vi "DAQ - 567 Modules - SubVI.vi"(11 "array":dbl[](array[numeric])) -> (3 "output array":dbl[](array[numeric]))   [LabVIEW 2013]
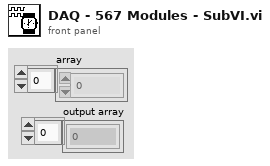
[diagram p1: front panel]
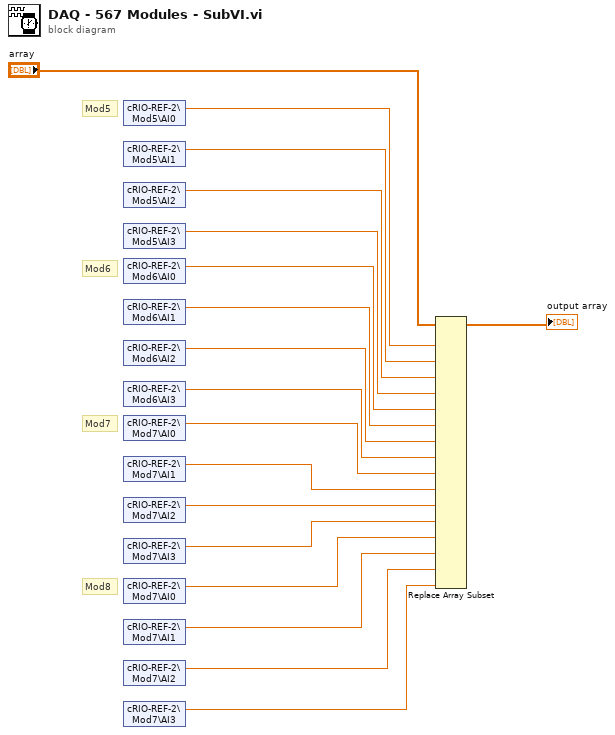
[diagram p0: block diagram]
diagram:
  # "Mod8"
  # "Mod7"
  # "Mod6"
  # "Mod5"
  n1 = shared-variable "cRIO-REF-2\\Mod5\\AI0"() -> (w18:dbl)  [unwired: 1 in, 1 out]
  n2 = shared-variable "cRIO-REF-2\\Mod5\\AI1"() -> (w17:dbl)  [unwired: 1 in, 1 out]
  n3 = shared-variable "cRIO-REF-2\\Mod5\\AI2"() -> (w16:dbl)  [unwired: 1 in, 1 out]
  n4 = shared-variable "cRIO-REF-2\\Mod5\\AI3"() -> (w15:dbl)  [unwired: 1 in, 1 out]
  n5 = shared-variable "cRIO-REF-2\\Mod6\\AI0"() -> (w14:dbl)  [unwired: 1 in, 1 out]
  n6 = shared-variable "cRIO-REF-2\\Mod6\\AI1"() -> (w13:dbl)  [unwired: 1 in, 1 out]
  n7 = shared-variable "cRIO-REF-2\\Mod6\\AI2"() -> (w12:dbl)  [unwired: 1 in, 1 out]
  n8 = shared-variable "cRIO-REF-2\\Mod6\\AI3"() -> (w11:dbl)  [unwired: 1 in, 1 out]
  n9 = shared-variable "cRIO-REF-2\\Mod7\\AI0"() -> (w10:dbl)  [unwired: 1 in, 1 out]
  n10 = shared-variable "cRIO-REF-2\\Mod7\\AI1"() -> (w9:dbl)  [unwired: 1 in, 1 out]
  n11 = shared-variable "cRIO-REF-2\\Mod7\\AI2"() -> (w8:dbl)  [unwired: 1 in, 1 out]
  n12 = shared-variable "cRIO-REF-2\\Mod7\\AI3"() -> (w7:dbl)  [unwired: 1 in, 1 out]
  n13 = shared-variable "cRIO-REF-2\\Mod7\\AI0"() -> (w4:dbl)  [unwired: 1 in, 1 out]
  n14 = shared-variable "cRIO-REF-2\\Mod7\\AI1"() -> (w3:dbl)  [unwired: 1 in, 1 out]
  n15 = shared-variable "cRIO-REF-2\\Mod7\\AI2"() -> (w2:dbl)  [unwired: 1 in, 1 out]
  n16 = shared-variable "cRIO-REF-2\\Mod7\\AI3"() -> (w1:dbl)  [unwired: 1 in, 1 out]
  n17 = Replace Array Subset(array="array", new element #1=w18, new element #2=w17, new element #3=w16, new element #4=w15, new element #5=w14, new element #6=w13, new element #7=w12, new element #8=w11, new element #9=w10, new element #10=w9, new element #11=w8, new element #12=w7, new element #13=w4, new element #14=w3, new element #15=w2, new element #16=w1) -> (→"output array":dbl[])  [unwired: 16 in]
